vi "External Interface - Set Value.vi"(0 "VI Name":path, 1 "Control Name":string, 3 "String Control Value":string, 4 "Variant Control Value":variant, 5 "error in":errorcluster, 7 "Machine Name":string) -> (17 "Return Message":string, 19 "error out":errorcluster)   [LabVIEW 2010]
uses:
  Utilities/Error Log.llb/Error Log - Priority.ctl
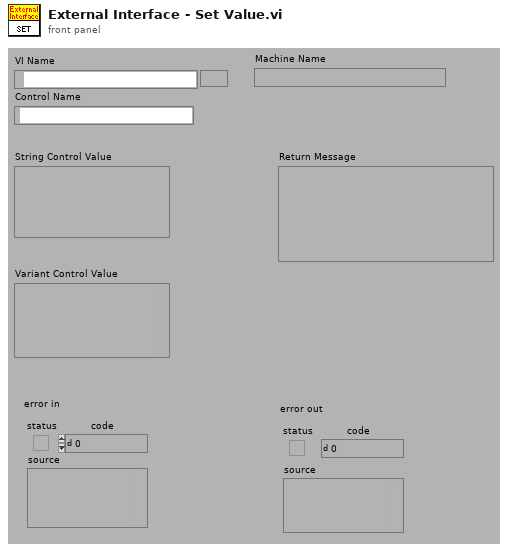
[diagram p1: front panel]
types:
  T1 = enum16{"Create Queue", "Get Queue Ref", "Add to Queue", "Close Queue"}
  T2 = typedef "Error Log - Priority.ctl" = enum16{"None", "Log", "SECI and Log"}
  T3 = enum32{"Bad", "Idle", "Run top level", "Running"}
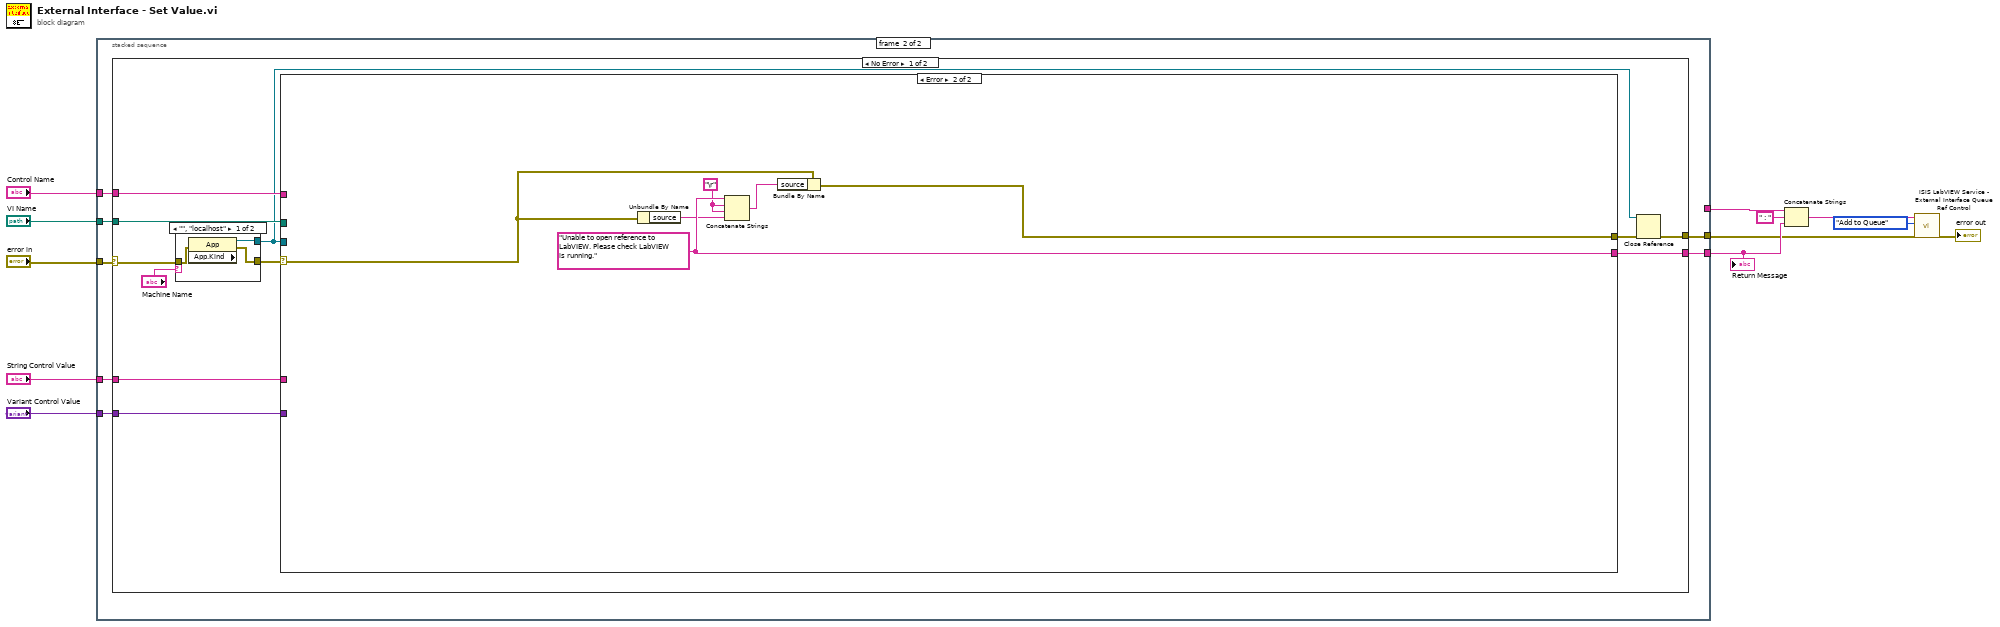
[diagram p0: block diagram]
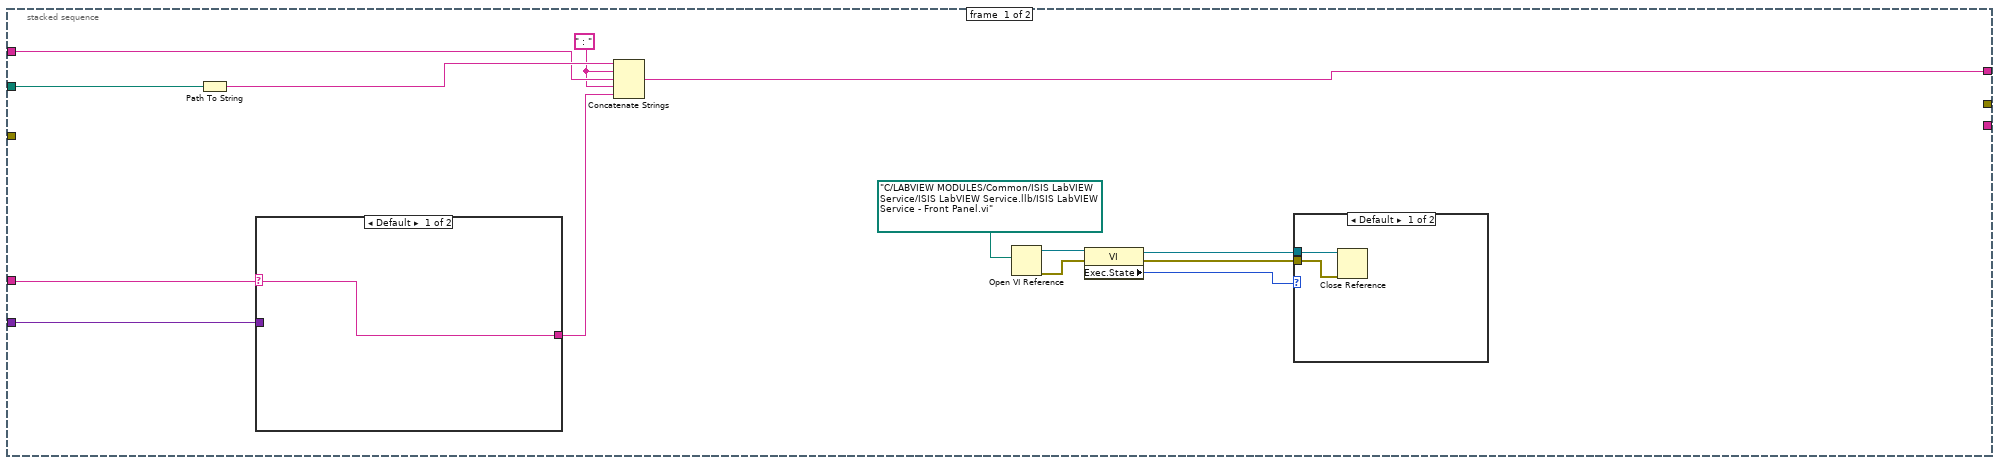
[diagram p2: hidden frame]
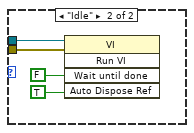
[diagram p3: hidden frame]
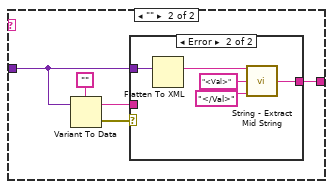
[diagram p4: hidden frame]
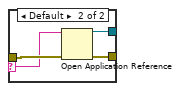
[diagram p6: hidden frame]
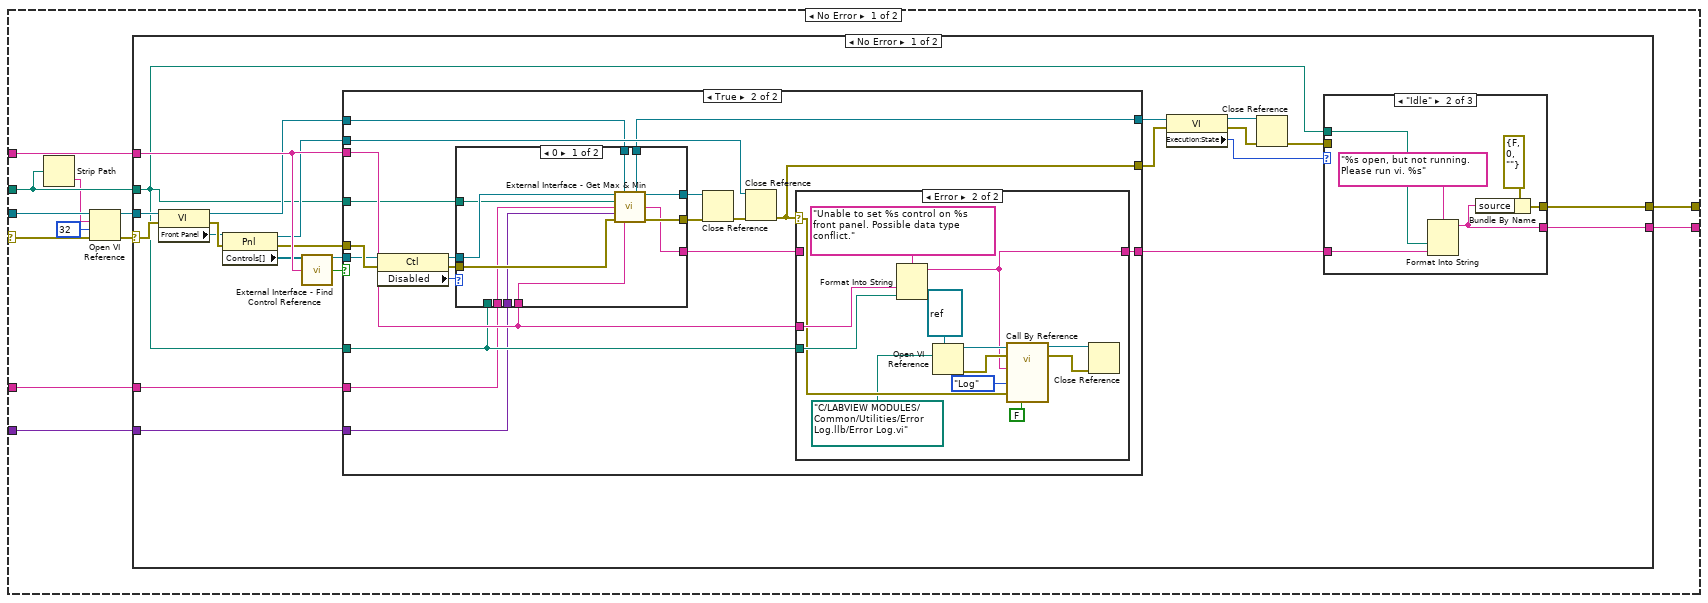
[diagram p7: hidden frame]
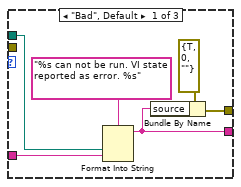
[diagram p8: hidden frame]
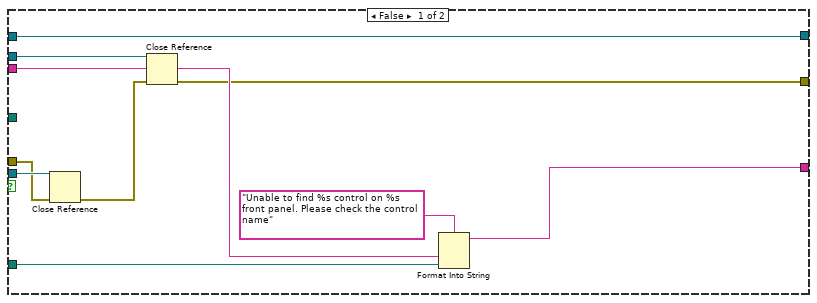
[diagram p10: hidden frame]
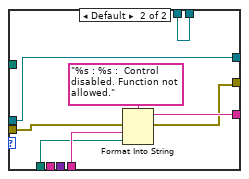
[diagram p11: hidden frame]
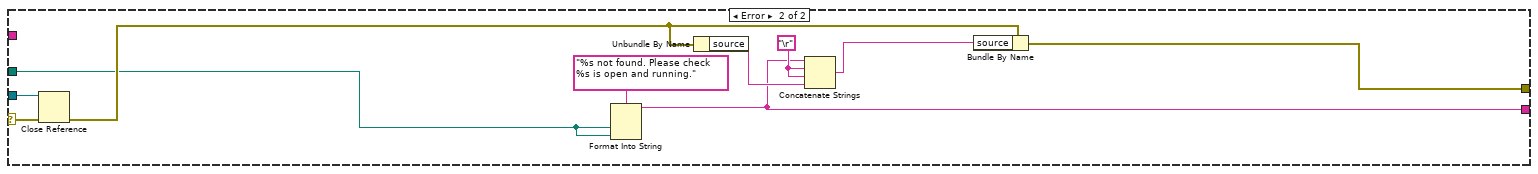
[diagram p13: hidden frame]
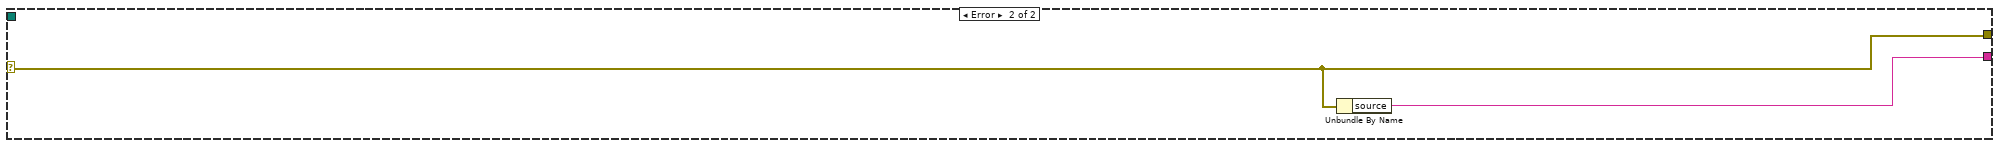
[diagram p14: hidden frame]
diagram:
  n1 = stacked-sequence {
    tunnel: [_ w51] -> w6
    tunnel: "error in" -> [_ w50]
    tunnel: [_ w49] -> w4
    tunnel: "VI Name" -> [w26 w48]
    tunnel: "Control Name" -> [w24 w47]
    tunnel: "String Control Value" -> [w22 w46]
    tunnel: "Variant Control Value" -> [w21 w45]
    tunnel: [w19 _] -> w7
    frame #0 {
      w23 = " : "
      n2 = Path To String(path=w26) -> (string=w25:string)
      n3 = case shown="Default" w22 {
        selector: w22 -> [w33 _]
        tunnel: w21 -> [_ w37]
        tunnel: [w33 w38] -> w20
        frame Default {
        }
        frame "" {
          n4 = Variant To Data(Variant=w37, type="") -> (error out=w35:errorcluster, data=w34:string)  [unwired: 1 in]
          n5 = case shown="Error" w35 {
            tunnel: w37 -> [_ w44]
            tunnel: [w39 w42] -> w38
            tunnel: w34 -> [w39 _]
            frame No Error {
            }
            frame Error {
              n6 = Flatten To XML(anything=w44) -> (xml string=w43:string)
              n7 = call "String - Extract Mid String.vi"("String"=w43, "Start search string"="<Val>", "End search string"="</Val>" ("Start search string")) -> ("String - Middle"=w42:string)  [unwired: 6 in, 6 out]
            }
          }
        }
      }
      n8 = Concatenate Strings(w25, w23, w24, w23, w20) -> (w19:string)
      n9 = Open VI Reference(vi path=path "C:/LABVIEW MODULES/Common/ISIS LabVIEW Service/ISIS LabVIEW Service.llb/ISIS LabVIEW Service - Front Panel.vi") -> (vi reference=w17:refnum<vi>, error out=w16:errorcluster)  [unwired: 5 in]
      n10 = property class="VI"(reference=w17, error in=w16) -> (reference out=w15:refnum<vi>, error out=w14:errorcluster, "Exec.State"=w13:T3)
      n11 = case shown="Default" w13 {
        tunnel: w15 -> [w28 w30]
        tunnel: w14 -> [w27 w29]
        frame Default {
          n12 = Close Reference(reference=w28, error in (no error)=w27) -> ()  [unwired: 1 out]
        }
        frame "Idle" {
          n13 = invoke class="VI" method="Run VI"(reference=w30, error in=w29, "Wait until done"=FALSE ("Wait Until Done"), "Auto Dispose Ref"=TRUE ("Wait Until Done")) -> ()  [unwired: 1 in, 5 out]
        }
      }
    }
    frame #1 {
      n14 = case shown="No Error" w50 {
        selector: w50 -> [w60 w198]
        tunnel: [w61 w197] -> w51
        tunnel: [w54 w198] -> w49
        tunnel: w48 -> [w59 _]
        tunnel: w47 -> [w58 _]
        tunnel: w46 -> [w57 _]
        tunnel: w45 -> [w56 _]
        frame No Error {
          n15 = case shown="\"\", \"localhost\"" "Machine Name" {
            selector: "Machine Name" -> [_ w66]
            tunnel: [w64 w69] -> w62
            tunnel: w60 -> [w63 w68]
            tunnel: [w65 w67] -> w53
            frame "", "localhost" {
              n16 = property class="App" props=["App.Kind"](error in=w63) -> (reference out=w65:refnum<vi>, error out=w64:errorcluster)  [unwired: 1 in, 1 out]
            }
            frame Default {
              n17 = Open Application Reference(8:w68, 11:w66) -> (0:w69:errorcluster, 3:w67:refnum<vi>)  [unwired: 2 in]
            }
          }
          n18 = case shown="Error" w62 {
            selector: w62 -> [w79 w191]
            tunnel: w53 -> [w81 _]
            tunnel: [w77 w196] -> w61
            tunnel: [w76 w192] -> w55
            tunnel: w59 -> [w72 _]
            tunnel: w58 -> [w75 _]
            tunnel: w57 -> [w74 _]
            tunnel: w56 -> [w73 _]
            frame No Error {
              n19 = Strip Path(path=w72) -> (name=w71:string)  [unwired: 1 out]
              n20 = Open VI Reference(application reference (local)=w81, vi path=w71, options=32, error in (no error)=w79) -> (vi reference=w80:refnum<vi>, error out=w78:errorcluster)  [unwired: 2 in]
              n21 = case shown="No Error" w78 {
                selector: w78 -> [w100 w183]
                tunnel: w80 -> [w101 w184]
                tunnel: [w83 w186] -> w77
                tunnel: [w87 w185] -> w76
                tunnel: w75 -> [w104 _]
                tunnel: w74 -> [w103 _]
                tunnel: w73 -> [w102 _]
                tunnel: w72 -> [w82 w181]
                frame No Error {
                  n22 = property class="VI"(reference=w101, error in=w100) -> (reference out=w96:refnum<vi>, error out=w99:errorcluster, "Front Panel"=w97:refnum<vi>)
                  n23 = property class="Pnl"(reference=w97, error in=w99) -> (reference out=w98:refnum<vi>, error out=w95:errorcluster, "Controls[]"=w94:refnum<vi>[])
                  n24 = call "External Interface - Find Control Reference.vi"("Control References - Top Level"=w94, "Control Name"=w104) -> ("Ctl Refnum"=w92:refnum<vi>, "Found"=w93:bool)  [unwired: 11 in, 1 out]
                  n25 = case shown="True" w93 {
                    tunnel: w82 -> [w126 w135]
                    tunnel: [w125 w147] -> w84
                    tunnel: w95 -> [w120 w140]
                    tunnel: w104 -> [w127 w142]
                    tunnel: w98 -> [w123 w146]
                    tunnel: w96 -> [w124 w143]
                    tunnel: [w122 w130] -> w90
                    tunnel: w103 -> [_ w134]
                    tunnel: w102 -> [_ w133]
                    tunnel: w92 -> [w121 w132]
                    tunnel: [w124 w131] -> w91
                    tunnel: w82 -> [_ w129]
                    frame False {
                      n26 = Close Reference(reference=w121, error in (no error)=w120) -> (error out=w119:errorcluster)
                      n27 = Close Reference(reference=w123, error in (no error)=w119) -> (error out=w122:errorcluster)
                      n28 = Format Into String(format string="Unable to find %s control on %s front panel. Please check the control name", w127, w126) -> (resulting string=w125:string)  [unwired: 2 in, 1 out]
                    }
                    frame True {
                      n29 = property class="Ctl"(reference=w132, error in=w140) -> (reference out=w138:refnum<vi>, error out=w139:errorcluster, "Disabled"=w137:u8)
                      n30 = case shown="0" w137 {
                        tunnel: [w158 w165] -> w144
                        tunnel: w143 -> [w157 w166]
                        tunnel: [w156 w166] -> w131
                        tunnel: w142 -> [w155 w163]
                        tunnel: [w154 w159] -> w141
                        tunnel: w139 -> [w153 w160]
                        tunnel: w138 -> [w152 w165]
                        tunnel: [w149 w162] -> w136
                        tunnel: w135 -> [_ w161]
                        tunnel: w134 -> [w151 _]
                        tunnel: w133 -> [w150 _]
                        tunnel: w129 -> [w148 _]
                        frame 0 {
                          n31 = call "External Interface - Get Max & Min.vi"("Ctl Refnum In"=w152, "VI Refnum In"=w157, "VI Name"=w148, "String Control Value"=w151, "Variant Control Value"=w150, "error in"=w153, "Control Name"=w155) -> ("VI Refnum Out"=w156:refnum<vi>, "Ctl Refnum Out"=w158:refnum<vi>, "Message"=w149:string, "error out"=w154:errorcluster)  [unwired: 5 in]
                        }
                        frame Default {
                          n32 = Format Into String(format string="%s : %s :  Control disabled. Function not allowed.", error in=w160, w163, w161) -> (resulting string=w162:string, error out=w159:errorcluster)  [unwired: 1 in]
                        }
                      }
                      n33 = Close Reference(reference=w144, error in (no error)=w141) -> (error out=w145:errorcluster)
                      n34 = Close Reference(reference=w146, error in (no error)=w145) -> (error out=w130:errorcluster)
                      n35 = case shown="Error" w130 {
                        selector: w130 -> [_ w170]
                        tunnel: [w167 w168] -> w147
                        tunnel: w142 -> [_ w179]
                        tunnel: w135 -> [_ w178]
                        tunnel: w136 -> [w167 _]
                        frame No Error {
                        }
                        frame Error {
                          n36 = Format Into String(format string="Unable to set %s control on %s front panel. Possible data type conflict.", w179, w178) -> (resulting string=w168:string)  [unwired: 2 in, 1 out]
                          n37 = Open VI Reference(type specifier VI Refnum (for type only)=refnum<vi> refnum, vi path=path "C:/LABVIEW MODULES/Common/Utilities/Error Log.llb/Error Log.vi") -> (vi reference=w171:refnum<vi>, error out=w172:errorcluster)  [unwired: 4 in]
                          n38 = call-by-ref "?"(reference=w171, error in=w172, "Error log message"=w168, "Priority"=Error_Log_-_Priority."Log", "error in (no error)"=w170, "Disconnecting"=FALSE) -> (reference out=w173:refnum<vi>, error out=w174:errorcluster)  [unwired: 11 in, 1 out]
                          n39 = Close Reference(reference=w173, error in (no error)=w174) -> ()  [unwired: 1 out]
                        }
                      }
                    }
                  }
                  n40 = property class="VI"(reference=w91, error in=w90) -> (reference out=w88:refnum<vi>, error out=w89:errorcluster, "Execution:State"=w85:T3)
                  n41 = Close Reference(reference=w88, error in (no error)=w89) -> (error out=w86:errorcluster)
                  n42 = case shown="\"Idle\"" w85 {
                    tunnel: [w108 w114 w117] -> w83
                    tunnel: [w107 w113 w118] -> w87
                    tunnel: w86 -> [_ _ w118]
                    tunnel: w84 -> [w105 w111 w117]
                    tunnel: w82 -> [w106 w112 _]
                    frame "Bad", Default {
                      n43 = Format Into String(format string="%s can not be run. VI state reported as error. %s", w106, w105) -> (resulting string=w108:string)  [unwired: 2 in, 1 out]
                      n44 = Bundle By Name(cluster=errorcluster {"status"=TRUE, "code"=0, "source"=""} ("error out"), "source"=w108) -> (w107:errorcluster)
                    }
                    frame "Idle" {
                      n45 = Format Into String(format string="%s open, but not running. Please run vi. %s", w112, w111) -> (resulting string=w114:string)  [unwired: 2 in, 1 out]
                      n46 = Bundle By Name(cluster=errorcluster {"status"=FALSE, "code"=0, "source"=""} ("error out"), "source"=w114) -> (w113:errorcluster)
                    }
                    frame "Run top level", "Running" {
                    }
                  }
                }
                frame Error {
                  w187 = "\r"
                  n47 = Close Reference(reference=w184, error in (no error)=w183) -> (error out=w182:errorcluster)
                  n48 = Format Into String(format string="%s not found. Please check %s is open and running.", w181, w181) -> (resulting string=w186:string)  [unwired: 2 in, 1 out]
                  n49 = Unbundle By Name(w182) -> ("source"=w188:string)
                  n50 = Concatenate Strings(w186, w187, w187, w188) -> (w189:string)
                  n51 = Bundle By Name(cluster=w182, "source"=w189) -> (w185:errorcluster)
                }
              }
            }
            frame Error {
              w193 = "\r"
              w196 = "Unable to open reference to LabVIEW. Please check LabVIEW is running."
              n52 = Unbundle By Name(w191) -> ("source"=w194:string)
              n53 = Concatenate Strings(w196, w193, w193, w194) -> (w195:string)
              n54 = Bundle By Name(cluster=w191, "source"=w195) -> (w192:errorcluster)
            }
          }
          n55 = Close Reference(reference=w53, error in (no error)=w55) -> (error out=w54:errorcluster)
        }
        frame Error {
          n56 = Unbundle By Name(w198) -> ("source"=w197:string)
        }
      }
    }
  }
  "Return Message" <- w6
  n57 = Concatenate Strings(w7, " : ", w6) -> (w3:string)
  n58 = call "ISIS LabVIEW Service - External Interface Queue Ref Control.vi"("error in (no error)"=w4, "Action"=T1."Add to Queue", "External Interface Message"=w3) -> ("error out"=→"error out":errorcluster)  [unwired: 7 in, 1 out]
